vi "Stop Core.vi"(10 "final error code":i32, 11 "Node Guard in":refnum<class "Node Guard.lvclass">) -> (3 "Node Guard out":refnum<class "Node Guard.lvclass">)   [LabVIEW 2020, in "CANopen.lvlib" / "Network Management.lvlib" / "Node Guard.lvlib" / "Node Guard.lvclass"]
doc: "<p>(<strong>Filename</strong>: <span class=\"dnl\">Actor Framework.lvlib:Actor.lvclass:Stop Core.vi</span>)</p>\n<p>Defines what the actor does before it stops. Use the <strong>final error code</strong> input to determine whether the actor shut down in response to an error.</p>\n<p>By default, this method passes the Stop message along to all <a href=\"nihelplauncher://docs/csh?context=lvcore_lvcomm_af_launch_nested_actor\">auto-stop nested actors</a>. A descendant class may override this method to define additional behavior, such as shutting down any processes the actor initiated in its override of the <a href=\"nihelplauncher://docs/csh?context=lvcore_lvcomm_af_actor_core\">Actor Core</a> method.</p>"
uses:
  Node Guard.lvclass
  Node Guard.lvclass/Node Guard.ctl
  <vilib>/ActorFramework/Actor/Actor.lvclass
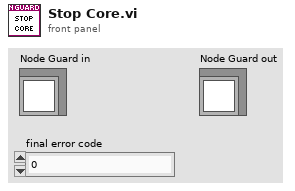
[diagram p1: front panel]
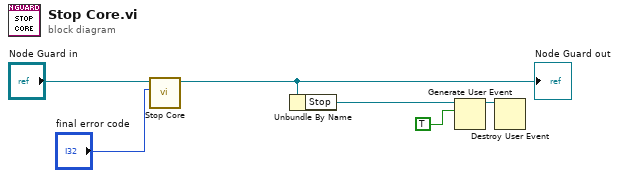
[diagram p0: block diagram]
diagram:
  n1 = call-parent "Stop Core.vi"("final error code"="final error code", "Actor in"="Node Guard in") -> ("Actor out"=w4:refnum<class "Node Guard.lvclass">)  [unwired: 9 in]
  "Node Guard out" <- w4
  n2 = Unbundle By Name(w4) -> ("Stop"=w3:refnum<user-event>)
  n3 = Generate User Event(user event=w3, event data cluster=TRUE ("event data")) -> (user event out=w2:refnum<user-event>)  [unwired: 2 in, 1 out]
  n4 = Destroy User Event(user event=w2) -> ()  [unwired: 1 in, 1 out]
